vi "Field_Rotation_Test.vi"() -> ()   [LabVIEW 2011]
panel:
  out "RA Tel":dbl=70342.56719999999 caption="Asc. Droite" format="%<%H:%M:%S%1u>t"
  out "DEC Tel":dbl=35996.6916 caption="Déclinaison" format="%<%H:%M:%S%0u>t"
  out "Rotation":dbl=90.0 min=-120.0 max=120.0 step=1.0 format="%.1f"
  in  "CentreTel X":i32=648675 min=1 max=1000000
  in  "CentreTel Y":i32=37988 max=1000000
  out "arcsec/pulse":dbl=5.45268e-05 format="%.5e"
  out "FOV":dbl format="%.1f"
  in  "OffrotChamp":dbl=300.0 format="%.2f"
  in  "Reference X":i32=669353 min=0 max=1000000
  in  "Reference Y":i32=53562 min=0 max=1000000
  out "TableXYPos":cluster{dbl[], dbl[]}[](graph)
  out "Img RA":dbl=70342.56719999999 caption="ImgRA  [°]" format="%.6f"
  out "Img DEC":dbl=35996.6916 caption="ImgDEC  [°]" format="%.6f"
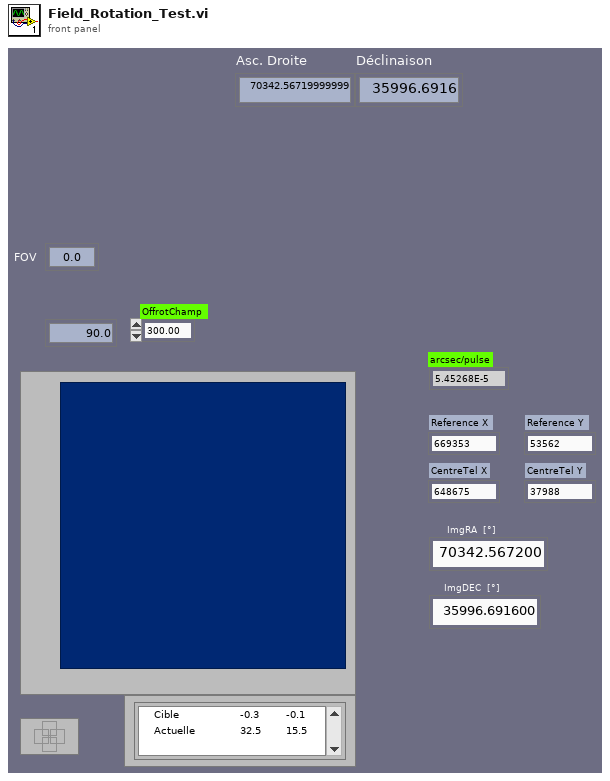
[diagram p1: front panel]
types:
  T1 = cluster{"NAXIS":dbl[], "CD":dbl[][], "CDELT":dbl[], "CRPIX":dbl[], "CTYPE":string[], "CRVAL":dbl[], "LONGPOLE":dbl, "LATPOLE":dbl, "PV2":dbl[]}
  T2 = typedef "LVRangeTypeDef.ctl" = cluster{"Minimum":dbl, "Maximum":dbl, "Increment":dbl, "Minor Increment":dbl, "Start":dbl}
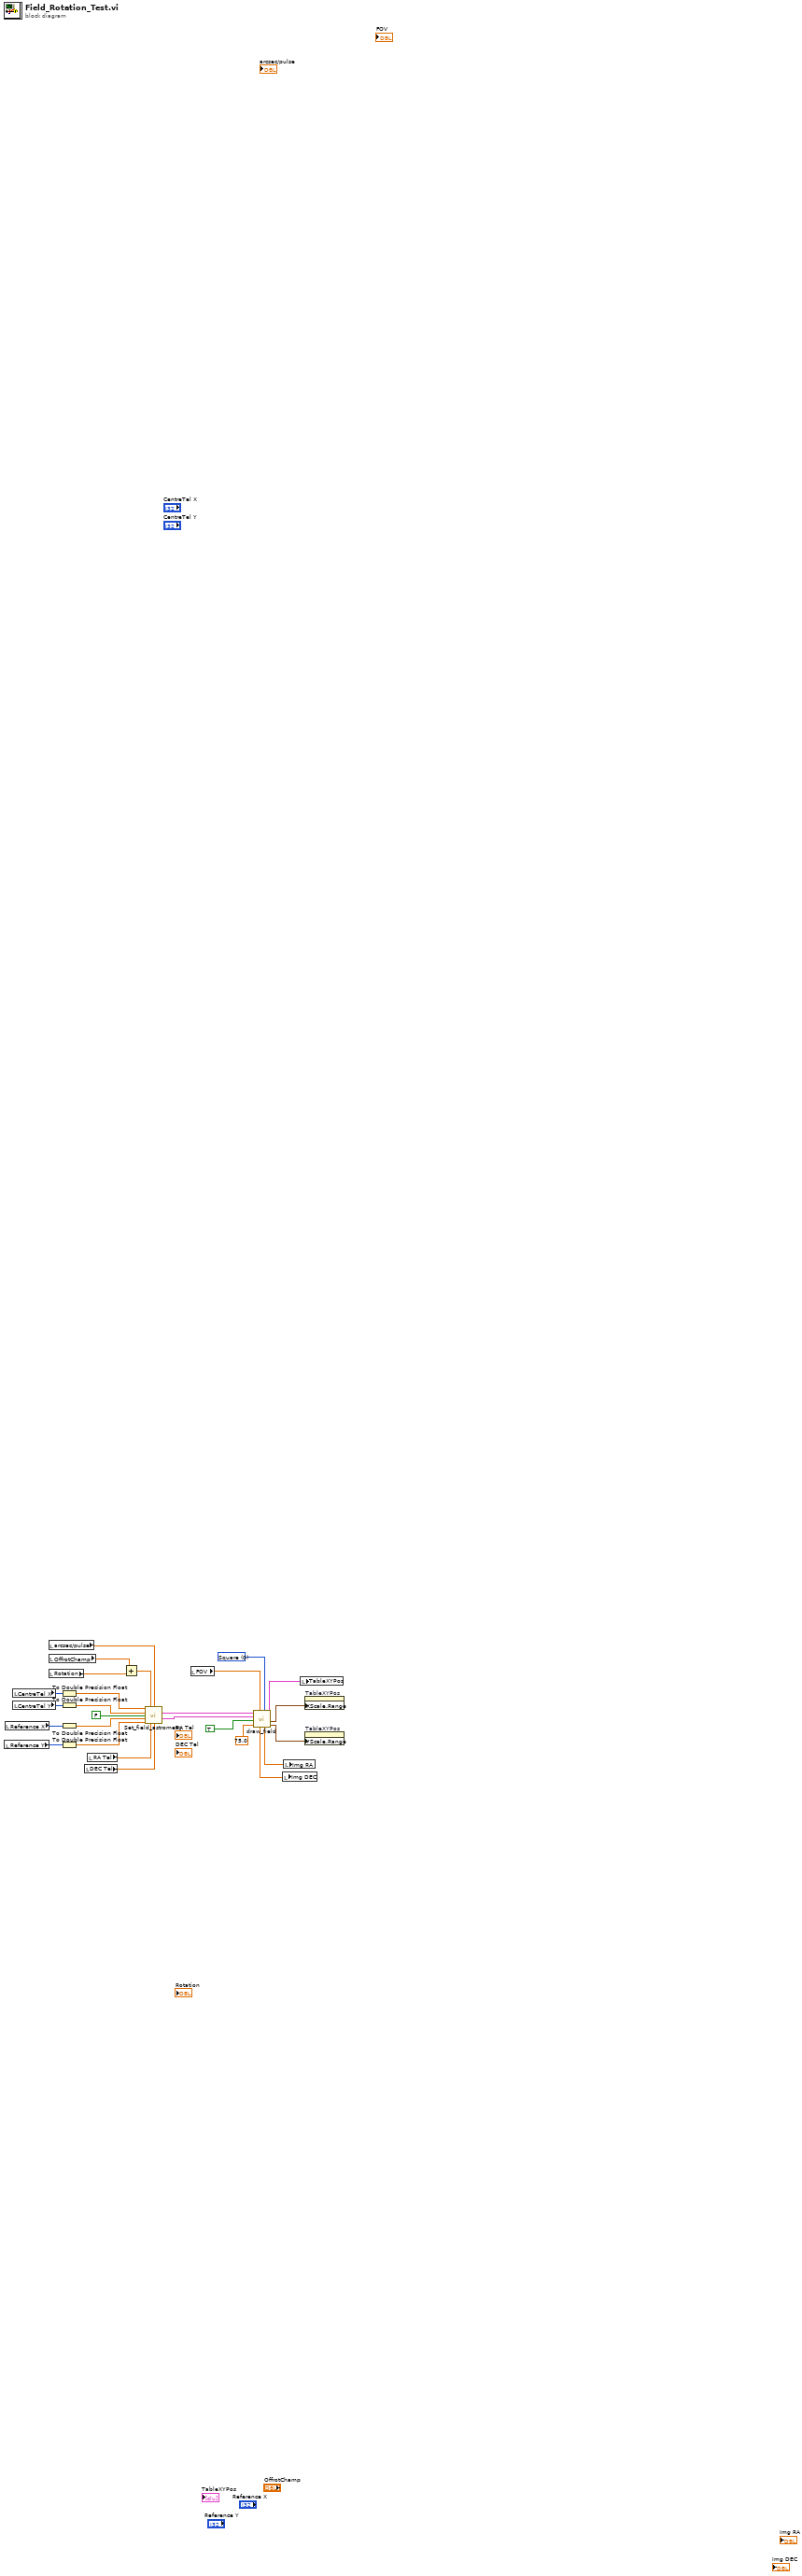
[diagram p0: block diagram]
diagram:
  w18 = u16 0 items=["Square", "Circle"] ("Ring")
  n1 = local read "Reference Y"() -> (w21:i32)
  n2 = local read "Reference X"() -> (w20:i32)
  n3 = local read "CentreTel X"() -> (w7:i32)
  n4 = local read "CentreTel Y"() -> (w10:i32)
  n5 = local read "arcsec/pulse"() -> (w16:dbl)
  n6 = local read "OffrotChamp"() -> (w19:dbl)
  n7 = local read "Rotation"() -> (w3:dbl)
  n8 = To Double Precision Float(number=w7) -> (double precision float=w8:dbl)
  n9 = To Double Precision Float(number=w10) -> (double precision float=w9:dbl)
  n10 = To Double Precision Float(number=w20) -> (double precision float=w6:dbl)
  n11 = To Double Precision Float(number=w21) -> (double precision float=w5:dbl)
  n12 = local read "DEC Tel"() -> (w12:dbl)
  n13 = local read "RA Tel"() -> (w11:dbl)
  n14 = Add(x=w19, y=w3) -> (x+y=w4:dbl)
  n15 = call "Set_field_astrometry.vi"("Cen x (pas)"=w8, "effective rotation (°)"=w4, "scale (\"/pas)"=w16, "Cen y (pas)"=w9, "Use Center?"=FALSE ("Ues Constant Size ?"), "Ref x (pas)"=w6, "Ref y (pas)"=w5, "RA (HH:MM:SS.S)"=w11, "DEC(DD:MM:SS)"=w12) -> ("Field Astrometry"=w24:T1, "Table Astrometry"=w23:T1)  [unwired: 5 in]
  n16 = local read "FOV"() -> (w17:dbl)
  n17 = call "draw_field.vi"("Ring"=w18, "FOV"=w17, "margin/size"=75.0, "Ues Constant Size ?"=TRUE, "Table_Astrometry"=w23, "Field_Astrometry"=w24) -> ("Y Scale.Range"=w2:T2, "X Scale.Range"=w1:T2, "TableXYPos"=w22:cluster{dbl[], dbl[]}[], "ImgRA"=w25:dbl, "ImgDEC"=w26:dbl)  [unwired: 1 in]
  n18 = local write "Img DEC"(w26) -> ()
  n19 = local write "Img RA"(w25) -> ()
  n20 = local write "TableXYPos"(w22) -> ()
  n21 = property on="TableXYPos" class="XYGraph (strict)"("XScale.Range"=w1) -> ()  [unwired: 2 in, 2 out]
  n22 = property on="TableXYPos" class="XYGraph (strict)"("YScale.Range"=w2) -> ()  [unwired: 2 in, 2 out]
